vi "TranslateMe.vi"() -> ()   [LabVIEW 2017]
panel:
  in  "Cluster":T1 caption="Tros"
  out "Array":string[](array[string]) caption="Reeks"
  out "Waveform Chart":dbl(graph) caption="Golfvorm Grafiek"
  in  "Numeric":dbl caption="Engelse Onderschrift"
  in  "String":string caption="Engelse Onderschrift"
  in  "Boolean":bool caption="Engelse Onderschrift"
  # "This VI is used to test translation"
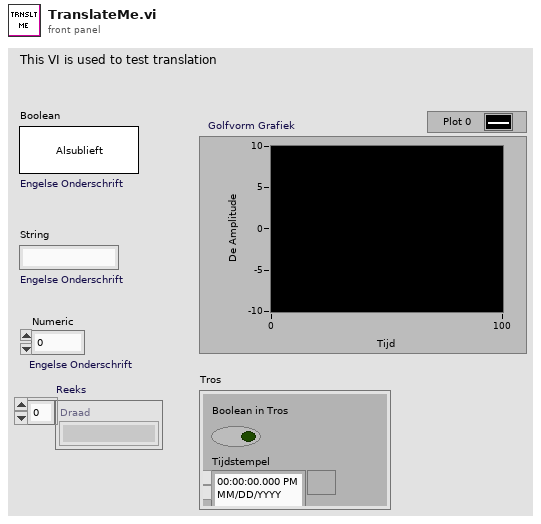
[diagram p1: front panel]
types:
  T1 = cluster{"Boolean in Cluster":bool, "Time Stamp":timestamp}
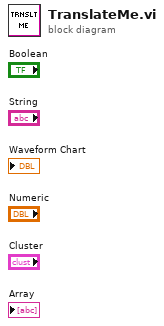
[diagram p0: block diagram]
diagram:
